vi "Get Attribute Tokens.vi"(11 "error":errorcluster) -> (1 "encoded":bool, 2 "array of JSON objects":T1[](array[typedef]), 3 "attribute tokens":cluster{"token type":T4, T2}[](array[cluster]))   [LabVIEW 2020, in "Multi Error Cluster.lvlib"]
doc: "Return the JSON token descriptor for the Attributes of the error cluster.\nAttribute tokens output will be empty if no section exists at all, and will have two entries for an empty attribute object."
uses:
  <vilib>/MultiError/TokenizeJSON/Multi Error Cluster.lvlib
  <vilib>/MultiError/TokenizeJSON/JSON Token Values.ctl
  <vilib>/MultiError/Errors Cluster Multiple Errors/JSON Token Descriptor.ctl
  <vilib>/MultiError/TokenizeJSON/JSON Raw Token Values.ctl
  <vilib>/MultiError/Errors Cluster Multiple Errors/JSON Object Descriptor.ctl
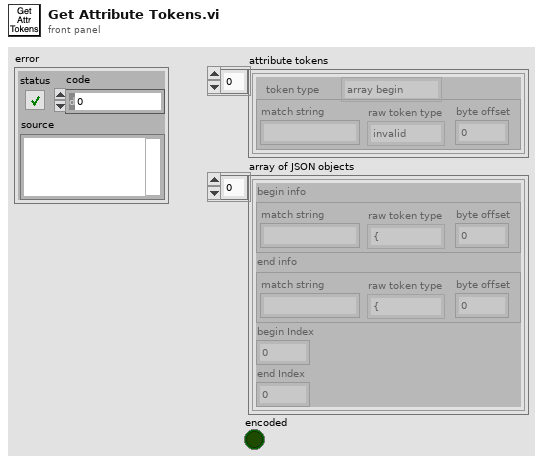
[diagram p1: front panel]
types:
  T1 = typedef "Multi Error Cluster.lvlib/JSON Object Descriptor.ctl" = cluster{"begin info":T2, "end info":T2, "begin Index":i32, "end Index":i32}
  T2 = typedef "Multi Error Cluster.lvlib/JSON Token Descriptor.ctl" = cluster{"match string":string, "raw token type":T3, "byte offset ":i32}
  T3 = typedef "Multi Error Cluster.lvlib/JSON Raw Token Values.ctl" = enum32{"{", "}", "[", "]", ",", ":", "\"", "number", "string", "true", "false", "null", "invalid"}
  T4 = typedef "Multi Error Cluster.lvlib/JSON Token Values.ctl" = enum32{"array begin", "array end", "object begin", "object end", "value", "invalid", "name"}
  T5 = cluster{"whole match":string, "token index":i32}[]
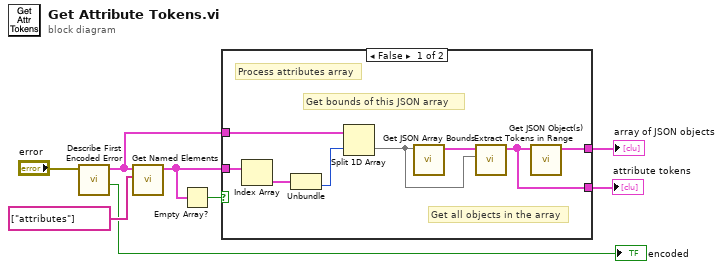
[diagram p0: block diagram]
diagram:
  n1 = call <vilib>:"Describe First Encoded Error.vi"("error in"="error") -> ("encoded"=→"encoded":bool, "tokens"=w7:cluster{"token type":T4, T2}[])  [unwired: 9 in]
  n2 = call <vilib>:"Get Named Elements.vi"("names"=string[] ["attributes"] ("Names"), "tokens"=w7) -> ("Found Token Info"=w3:T5)  [unwired: 9 in]
  n3 = Empty Array?(array=w3) -> (empty?=w2:bool)
  n4 = case shown="False" w2 {
    tunnel: w7 -> [w14 _]
    tunnel: w3 -> [w15 _]
    tunnel: [w11 _] -> w8
    tunnel: [w13 _] -> w1
    frame False {
      # "Get all objects in the array"
      # "Get bounds of this JSON array"
      # "Process attributes array"
      n5 = Index Array(array=w15) -> (element=w16:cluster{"whole match":string, "token index":i32})  [unwired: 1 in]
      n6 = Unbundle(w16) -> ("token index"=w12:i32)  [unwired: 1 out]
      n7 = Split 1D Array(array=w14, index=w12) -> (second subarray=w10:cluster{"token type":T4, T2}[])  [unwired: 1 out]
      n8 = call <vilib>:"Get JSON Array Bounds.vi"("tokens"=w10) -> ("array of JSON objects"=w9:T1[])  [unwired: 10 in]
      n9 = call <vilib>:"Extract Tokens in Range.vi"("tokens"=w10, "range info"=w9) -> ("tokens out"=w11:cluster{"token type":T4, "info":T2}[])  [unwired: 9 in]
      n10 = call <vilib>:"Get JSON Object(s).vi"("tokens"=w11) -> ("array of JSON objects"=w13:T1[])  [unwired: 10 in]
    }
    frame True {
    }
  }
  "attribute tokens" <- w8
  "array of JSON objects" <- w1
